vi "形态学处理 (子VI).vi"(11 "引用句柄输入":T1) -> (2 "Image Dst Out":T1, 3 "引用句柄输出":T1(plugin-control))   [LabVIEW 2012]
uses:
  <vilib>/vision/Image Controls.llb/IMAQ Image.ctl
  <vilib>/silver_ctls/ArrayMatrixCluster/Real Matrix NI_Silver.ctl
  <vilib>/vision/NI_Vision_Development_Module.lvlib
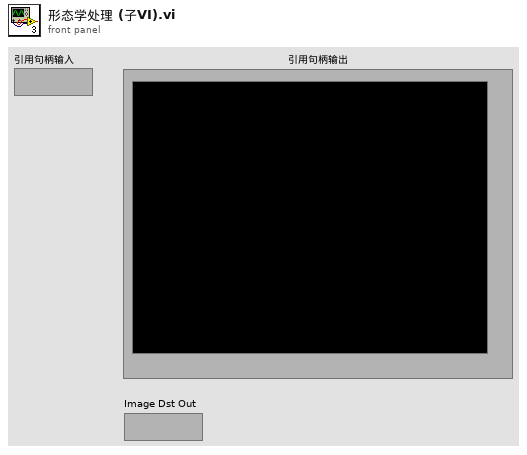
[diagram p1: front panel]
types:
  T1 = typedef "IMAQ Image.ctl" = refnum<image>
  T2 = typedef "Real Matrix NI_Silver.ctl" = u8[][]
  T3 = enum32{"AutoM", "Close", "Dilate", "Erode", "Gradient", "Gradient out", "Gradient in", "Hit miss", "Open", "PClose", "POpen", "Thick", "Thin"}
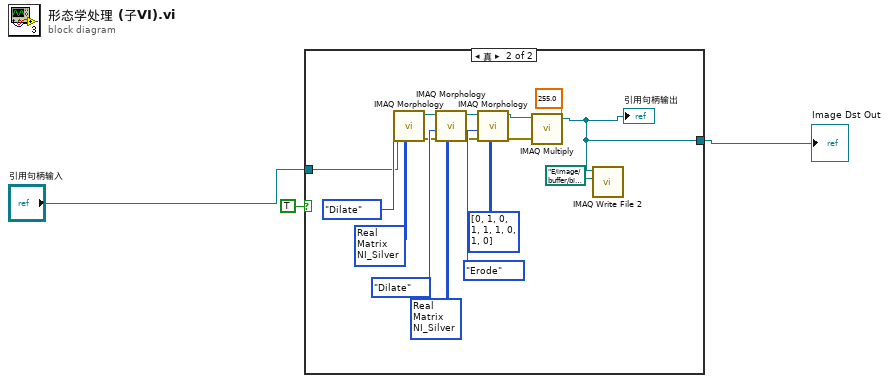
[diagram p0: block diagram]
diagram:
  n1 = case shown="真" TRUE {
    tunnel: [w4 w8] -> w2
    tunnel: "引用句柄输入" -> [w4 w9]
    frame False {
    }
    frame True {
      n2 = call "IMAQ Morphology"("Structuring Element"=T2 [[0, 0, 1, 0, 0], [0, 1, 1, 1, 0], [1, 1, 1, 1, 1], [0, 1, 1, 1, 0], [0, 0, 1, 0, 0]] ("腐蚀结构元素"), "Operation"=T3."Dilate", "Image Src"=w9) -> ("error out"=w7:errorcluster, "Image Dst Out"=w17:T1)  [unwired: 7 in]
      n3 = call "IMAQ Morphology"("Structuring Element"=T2 [[0, 0, 1, 0, 0], [0, 1, 1, 1, 0], [1, 1, 1, 1, 1], [0, 1, 1, 1, 0], [0, 0, 1, 0, 0]] ("膨胀结构元素 2"), "error in (no error)"=w7, "Operation"=T3."Dilate", "Image Src"=w17) -> ("error out"=w6:errorcluster, "Image Dst Out"=w16:T1)  [unwired: 6 in]
      n4 = call "IMAQ Morphology"("Structuring Element"=T2 [[0, 1, 0], [1, 1, 1], [0, 1, 0]] ("腐蚀结构元素"), "error in (no error)"=w6, "Operation"=T3."Erode", "Image Src"=w16) -> ("error out"=w5:errorcluster, "Image Dst Out"=w12:T1)  [unwired: 6 in]
      n5 = call "IMAQ Multiply"("Image Src A"=w12, "Constant"=sgl 255.0, "error in (no error)"=w5) -> ("Image Dst Out"=w8:T1)  [unwired: 4 in, 1 out]
      "引用句柄输出" <- w8
      n6 = call-poly "IMAQ Write File 2"("File Path"=path "E:/image/buffer/bin.bmp" ("二值图缓存"), "Image"=w8) -> ()  [unwired: 8 in, 2 out]
    }
  }
  "Image Dst Out" <- w2
